vi "farbanpassung geradeaus weiter.vi"(8 "error in (no error)":errorcluster caption="Fehler (Eingang, kein Fehler)", 11 "Device ID":T1(ring)) -> (0 "error out":errorcluster caption="Fehler (Ausgang)", 3 "Device ID Out":T1(ring))   [LabVIEW 2010]
uses:
  globale Variable 1.vi
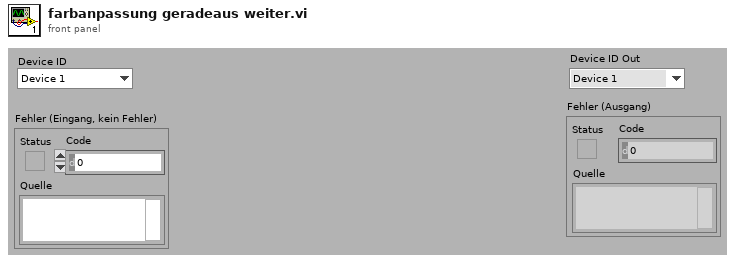
[diagram p1: front panel]
types:
  T1 = enum16{"Device 1", "Device 2", "Device 3", "Device 4", "Device 5", "Device 6", "Device 7", "Device 8"}
  T2 = enum8{"Robo Interface", "Extension 1", "Extension 2", "Extension 3"}
  T3 = enum8{"Output 1 (O1)", "Output 2 (O2)", "Output 3 (O3)", "Output 4 (O4)", "Output 5 (O5)", "Output 6 (O6)", "Output 7 (O7)", "Output 8 (O8)"}
  T4 = enum8{"Power 1", "Power 2", "Power 3", "Power 4", "Power 5", "Power 6", "Power 7", "Power 8"}
  T5 = enum8{"Goes High", "Goes Low", "Goes High or Low"}
  T6 = enum8{"Input 1 (I1)", "Input 2 (I2)", "Input 3 (I3)", "Input 4 (I4)", "Input 5 (I5)", "Input 6 (I6)", "Input 7 (I7)", "Input 8 (I8)"}
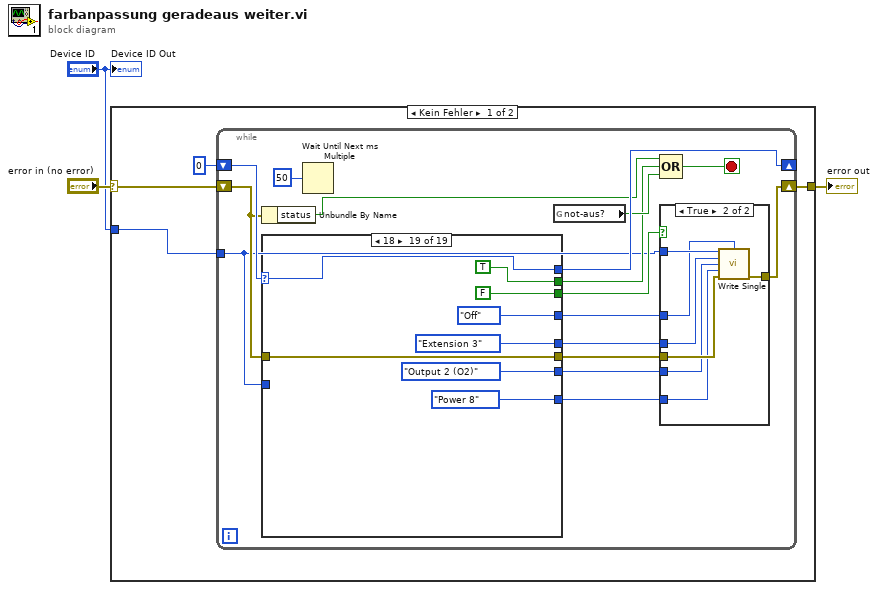
[diagram p0: block diagram]
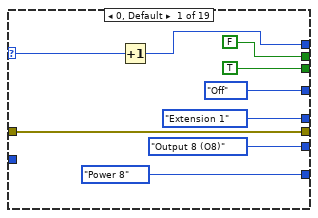
[diagram p3: hidden frame]
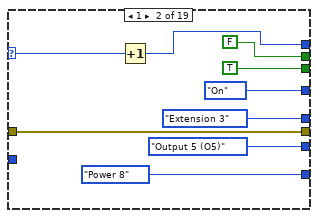
[diagram p4: hidden frame]
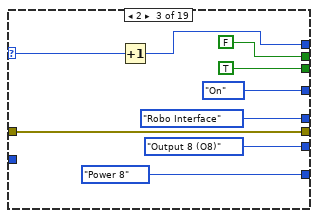
[diagram p5: hidden frame]
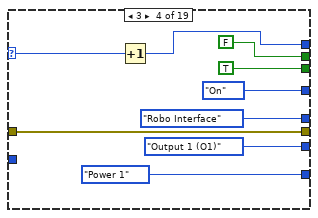
[diagram p6: hidden frame]
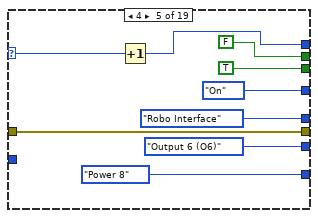
[diagram p7: hidden frame]
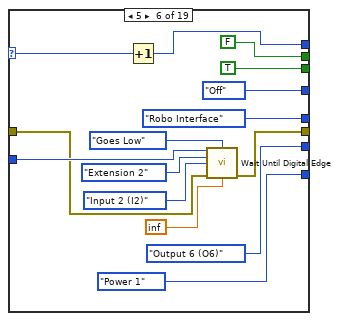
[diagram p8: hidden frame]
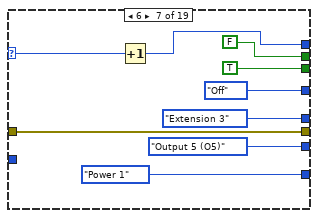
[diagram p9: hidden frame]
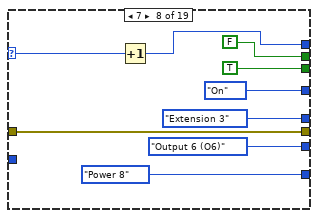
[diagram p10: hidden frame]
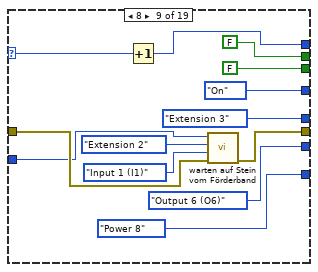
[diagram p11: hidden frame]
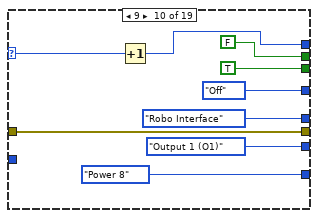
[diagram p12: hidden frame]
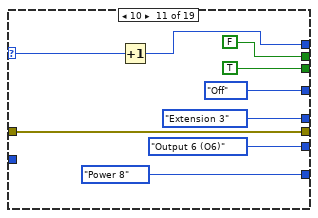
[diagram p13: hidden frame]
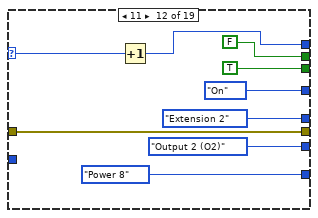
[diagram p14: hidden frame]
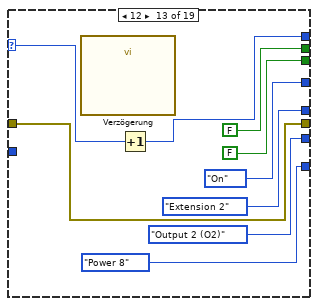
[diagram p15: hidden frame]
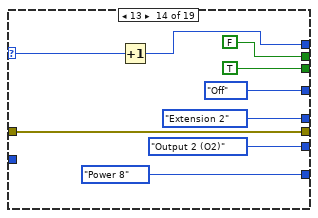
[diagram p16: hidden frame]
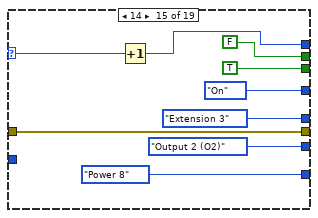
[diagram p17: hidden frame]
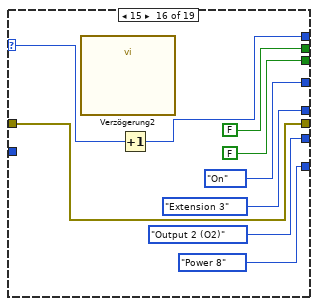
[diagram p18: hidden frame]
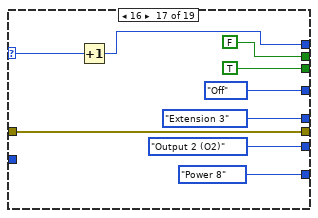
[diagram p19: hidden frame]
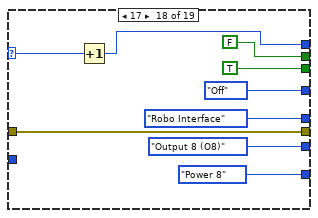
[diagram p20: hidden frame]
diagram:
  n1 = case shown="Kein Fehler" "error in (no error)" {
    selector: "error in (no error)" -> [w6 w212]
    tunnel: "Device ID" -> [w4 _]
    tunnel: [w5 w212] -> w1
    frame No Error {
      n2 = while {
        shift-right: [w21] -> _
        shift-left: 0 -> [w23]
        tunnel: w4 -> [w8]
        shift-right: [w17] -> w5
        shift-left: w6 -> [w16]
        stop <- w19 stop-if-true
        n3 = Unbundle By Name(w16) -> ("status"=w20:bool)
        n4 = case shown="18" w23 {
          selector: w23 -> [w39 w48 w57 w66 w75 w90 w99 w108 w121 w130 w139 w148 w157 w166 w175 w184 w193 w202 w204]
          tunnel: [TRUE TRUE TRUE TRUE TRUE TRUE TRUE TRUE FALSE TRUE TRUE TRUE FALSE TRUE TRUE FALSE TRUE TRUE FALSE] -> w22
          tunnel: [w38 w47 w56 w65 w74 w89 w98 w107 w120 w129 w138 w147 w156 w165 w174 w183 w192 w201 w204] -> w21
          tunnel: [w37 w46 w55 w64 w73 w79 w92 w101 w110 w123 w132 w141 w150 w159 w168 w177 w186 w195 w205] -> w18
          tunnel: w16 -> [w37 w46 w55 w64 w73 w80 w92 w101 w112 w123 w132 w141 w150 w159 w168 w177 w186 w195 w205]
          tunnel: [T2."Extension 1" ("Module") T2."Extension 3" ("Module") T2."Robo Interface" ("Module") T2."Robo Interface" ("Module") T2."Robo Interface" ("Module") T2."Robo Interface" ("Module") T2."Extension 3" ("Module") T2."Extension 3" ("Module") T2."Extension 3" ("Module") T2."Robo Interface" ("Module") T2."Extension 3" ("Module") T2."Extension 2" ("Module") T2."Extension 2" ("Module") T2."Extension 2" ("Module") T2."Extension 3" ("Module") T2."Extension 3" ("Module") T2."Extension 3" ("Module") T2."Robo Interface" ("Module") T2."Extension 3" ("Module")] -> w15
          tunnel: [T3."Output 8 (O8)" ("Single_Output") T3."Output 5 (O5)" ("Single_Output") T3."Output 8 (O8)" ("Single_Output") T3."Output 1 (O1)" ("Single_Output") T3."Output 6 (O6)" ("Single_Output") T3."Output 6 (O6)" ("Single_Output") T3."Output 5 (O5)" ("Single_Output") T3."Output 6 (O6)" ("Single_Output") T3."Output 6 (O6)" ("Single_Output") T3."Output 1 (O1)" ("Single_Output") T3."Output 6 (O6)" ("Single_Output") T3."Output 2 (O2)" ("Single_Output") T3."Output 2 (O2)" ("Single_Output") T3."Output 2 (O2)" ("Single_Output") T3."Output 2 (O2)" ("Single_Output") T3."Output 2 (O2)" ("Single_Output") T3."Output 2 (O2)" ("Single_Output") T3."Output 8 (O8)" ("Single_Output") T3."Output 2 (O2)" ("Single_Output")] -> w14
          tunnel: [T4."Power 8" ("Output_PWM") T4."Power 8" ("Output_PWM") T4."Power 8" ("Output_PWM") T4."Power 1" ("Output_PWM") T4."Power 8" ("Output_PWM") T4."Power 1" ("Output_PWM") T4."Power 1" ("Output_PWM") T4."Power 8" ("Output_PWM") T4."Power 8" ("Output_PWM") T4."Power 8" ("Output_PWM") T4."Power 8" ("Output_PWM") T4."Power 8" ("Output_PWM") T4."Power 8" ("Output_PWM") T4."Power 8" ("Output_PWM") T4."Power 8" ("Output_PWM") T4."Power 8" ("Output_PWM") T4."Power 8" ("Output_PWM") T4."Power 8" ("Output_PWM") T4."Power 8" ("Output_PWM")] -> w13
          tunnel: [enum8{"Off", "On"}."Off" ("Output_Action") enum8{"Off", "On"}."On" ("Output_Action") enum8{"Off", "On"}."On" ("Output_Action") enum8{"Off", "On"}."On" ("Output_Action") enum8{"Off", "On"}."On" ("Output_Action") enum8{"Off", "On"}."Off" ("Output_Action") enum8{"Off", "On"}."Off" ("Output_Action") enum8{"Off", "On"}."On" ("Output_Action") enum8{"Off", "On"}."On" ("Output_Action") enum8{"Off", "On"}."Off" ("Output_Action") enum8{"Off", "On"}."Off" ("Output_Action") enum8{"Off", "On"}."On" ("Output_Action") enum8{"Off", "On"}."On" ("Output_Action") enum8{"Off", "On"}."Off" ("Output_Action") enum8{"Off", "On"}."On" ("Output_Action") enum8{"Off", "On"}."On" ("Output_Action") enum8{"Off", "On"}."Off" ("Output_Action") enum8{"Off", "On"}."Off" ("Output_Action") enum8{"Off", "On"}."Off" ("Output_Action")] -> w12
          tunnel: [FALSE FALSE FALSE FALSE FALSE FALSE FALSE FALSE FALSE FALSE FALSE FALSE FALSE FALSE FALSE FALSE FALSE FALSE TRUE] -> w9
          tunnel: w8 -> [_ _ _ _ _ w83 _ _ w111 _ _ _ _ _ _ _ _ _ _]
          frame 0, Default {
            n5 = Increment(x=w39) -> (x+1=w38:i32)
          }
          frame 1 {
            n6 = Increment(x=w48) -> (x+1=w47:i32)
          }
          frame 2 {
            n7 = Increment(x=w57) -> (x+1=w56:i32)
          }
          frame 3 {
            n8 = Increment(x=w66) -> (x+1=w65:i32)
          }
          frame 4 {
            n9 = Increment(x=w75) -> (x+1=w74:i32)
          }
          frame 5 {
            n10 = Increment(x=w90) -> (x+1=w89:i32)
            n11 = call "Wait Until Digital Edge.vi"("Device ID"=w83, "Wait Until"=T5."Goes Low", "Module"=T2."Extension 2", "Digital_Input"=T6."Input 2 (I2)", "error in"=w80, "Time Out (10)"=inf) -> ("error out"=w79:errorcluster)  [unwired: 9 out]
          }
          frame 6 {
            n12 = Increment(x=w99) -> (x+1=w98:i32)
          }
          frame 7 {
            n13 = Increment(x=w108) -> (x+1=w107:i32)
          }
          frame 8 {
            n14 = Increment(x=w121) -> (x+1=w120:i32)
            n15 = call "warten auf Stein vom Förderband.vi"("error in (no error)"=w112, "Digital_Input"=T6."Input 1 (I1)", "Module"=T2."Extension 2", "Device ID"=w111) -> ("error out"=w110:errorcluster)  [unwired: 7 out]
          }
          frame 9 {
            n16 = Increment(x=w130) -> (x+1=w129:i32)
          }
          frame 10 {
            n17 = Increment(x=w139) -> (x+1=w138:i32)
          }
          frame 11 {
            n18 = Increment(x=w148) -> (x+1=w147:i32)
          }
          frame 12 {
            n19 = call "Verzögerung"() -> ()  [unwired: 2 in, 10 out]
            n20 = Increment(x=w157) -> (x+1=w156:i32)
          }
          frame 13 {
            n21 = Increment(x=w166) -> (x+1=w165:i32)
          }
          frame 14 {
            n22 = Increment(x=w175) -> (x+1=w174:i32)
          }
          frame 15 {
            n23 = call "Verzögerung2"() -> ()  [unwired: 2 in, 10 out]
            n24 = Increment(x=w184) -> (x+1=w183:i32)
          }
          frame 16 {
            n25 = Increment(x=w193) -> (x+1=w192:i32)
          }
          frame 17 {
            n26 = Increment(x=w202) -> (x+1=w201:i32)
          }
          frame 18 {
          }
        }
        n27 = Wait Until Next ms Multiple(millisecond multiple=50) -> ()  [unwired: 1 out]
        n28 = global read "globale Variable 1.vi" "not-aus?"() -> (w10:bool)
        n29 = Compound Arithmetic op=OR(w20, w9, w10) -> (w19:bool)
        n30 = case shown="TRUE" w22 {
          tunnel: w8 -> [_ w31]
          tunnel: w18 -> [w24 w30]
          tunnel: [w24 w29] -> w17
          tunnel: w15 -> [_ w28]
          tunnel: w14 -> [_ w27]
          tunnel: w13 -> [_ w26]
          tunnel: w12 -> [_ w25]
          frame False {
          }
          frame True {
            n31 = call "Write Single.vi"("Device ID"=w31, "Output_Action"=w25, "Module"=w28, "Single_Output"=w27, "Output_PWM"=w26, "error in"=w30) -> ("error out"=w29:errorcluster)  [unwired: 9 out]
          }
        }
      }
    }
    frame Error {
    }
  }
  "error out" <- w1
  "Device ID Out" <- "Device ID"
